vi "Drive Controller Interactive Check.vi"(8 "Interactive Command In":T1 {"Path stuff"."output cluster"."Limits"."StoopidFast (fps)" min=0.0; "Path stuff"."output cluster"."Limits"."Jerk (fps^3)" min=0.0 step=1.0; "Path stuff"."output cluster"."Limits"."Accel (fps^2)" min=0.0; "Path stuff"."output cluster"."Limits"."Velocity (fps)" min=0.0}, 9 "Default Command":T1 {"Path stuff"."output cluster"."Limits"."StoopidFast (fps)" min=0.0; "Path stuff"."output cluster"."Limits"."Jerk (fps^3)" min=0.0 step=1.0; "Path stuff"."output cluster"."Limits"."Accel (fps^2)" min=0.0; "Path stuff"."output cluster"."Limits"."Velocity (fps)" min=0.0}, 11 "Buttons":cluster{"Execute Cmd":bool, "Abort Cmd":bool}) -> (1 "Interactive Command Out":T1 {"Path stuff"."output cluster"."Limits"."StoopidFast (fps)" min=0.0; "Path stuff"."output cluster"."Limits"."Jerk (fps^3)" min=0.0 step=1.0; "Path stuff"."output cluster"."Limits"."Accel (fps^2)" min=0.0; "Path stuff"."output cluster"."Limits"."Velocity (fps)" min=0.0}, 2 "Trace String":string, 3 "Schedule":bool)   [LabVIEW 2019]
doc: "Check the Execute and Abort buttons and choose the data and trace string."
uses:
  Drive Setpoints.ctl
  Drive Operations.ctl
  bordeaux-pathinator/Bordeaux/Command Stuff/Single Cmd Info.ctl
  <vilib>/picture/picture.llb/imagedata.ctl
  bordeaux-pathinator/Bordeaux/Limits.ctl
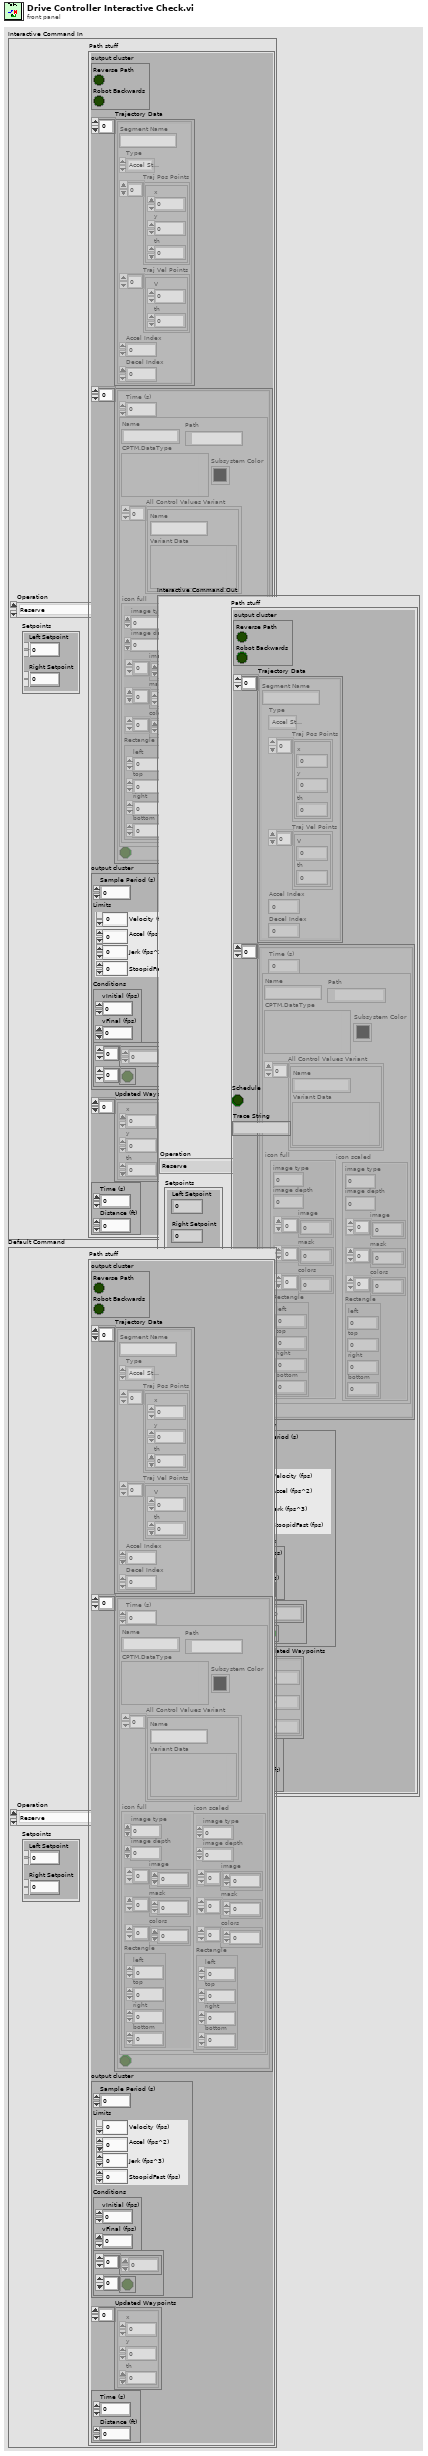
[diagram p1: front panel]
types:
  T1 = typedef "Drive Setpoints.ctl" = cluster{"Operation":T2, "Setpoints":cluster{"Left Setpoint":dbl, "Right Setpoint":dbl}, "Path stuff":cluster{"output cluster":cluster{"Reverse Path":bool, "Robot Backwards":bool}, "Trajectory Data":cluster{"Segment Name":string, "Type":enum16{"Accel Straight", "Const Straight", "Blend", "Circle"}, "Traj Pos Points":cluster{"x":dbl, "y":dbl, "th":dbl}[], "Traj Vel Points":cluster{"V":dbl, "th":dbl}[], "Accel Index":i32, "Decel Index":i32}[], cluster{"Time (s)":dbl, T3, bool}[], "output cluster":cluster{"Sample Period (s)":dbl, "Limits":T5, "Conditions":cluster{"vInitial (fps)":dbl, "vFinal (fps)":dbl}, cluster{dbl[], bool[]}}, "Updated Waypoints":cluster{"x":dbl, "y":dbl, "th":dbl}[], cluster{"Time (s)":dbl, "Distance (ft)":dbl}}}
  T2 = typedef "Drive Operations.ctl" = enum16{"Reserve", "Read Current", "Immediate", "Play Path"}
  T3 = typedef "Single Cmd Info.ctl" = cluster{"Name":string, "CPTM.DataType":variant, "All Control Values Variant":cluster{"Name":string, "Variant Data":variant}[], "icon full":T4, "icon scaled":T4, "Path":path, "Subsystem Color":u32}
  T4 = typedef "imagedata.ctl" = cluster{"image type":i32, "image depth":i32, "image":u8[], "mask":u8[], "colors":u32[], "Rectangle":cluster{"left":i16, "top":i16, "right":i16, "bottom":i16}}
  T5 = typedef "Limits.ctl" = cluster{"Velocity (fps)":dbl, "Accel (fps^2)":dbl, "Jerk (fps^3)":dbl, "StoopidFast (fps)":dbl}
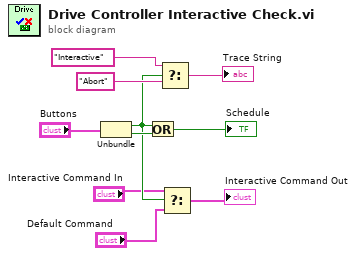
[diagram p0: block diagram]
diagram:
  n1 = Unbundle("Buttons") -> ("Execute Cmd"=w6:bool, "Abort Cmd"=w7:bool)
  n2 = Or(x=w6, y=w7) -> (x .or. y?=→"Schedule":bool)
  n3 = Select(t="Interactive", s=w6, f="Abort") -> (s? t:f=→"Trace String":string)
  n4 = Select(t="Interactive Command In", s=w6, f="Default Command") -> (s? t:f=→"Interactive Command Out":T1)
